vi "writeTiffFile.vi"(0 "Image Pixels (U16)":u16[][](array[numeric]), 1 "File Path":path) -> ()   [LabVIEW 2015]
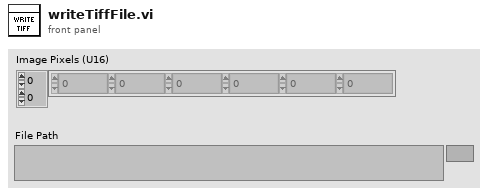
[diagram p1: front panel]
types:
  T1 = typedef "Image Type" = u32
  T2 = typedef "IMAQ Image.ctl" = refnum<image>
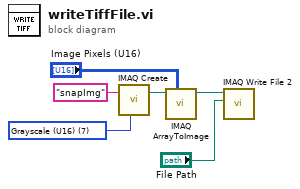
[diagram p0: block diagram]
diagram:
  w3 = T1 7 items=["Grayscale (U8)", "Grayscale (I16)", "Grayscale (SGL)", "Complex (CSG)", "RGB (U32)", "HSL (U32)", "RGB (U64)", "Grayscale (U16)"] ("Image Type")
  n1 = call "IMAQ Create"("Image Name"="snapImg", "Image Type"=w3) -> ("New Image"=w5:T2)  [unwired: 3 in, 1 out]
  n2 = call "IMAQ ArrayToImage"("Image Pixels (U16)"="Image Pixels (U16)", "Image"=w5) -> ("Image Out"=w6:T2)  [unwired: 8 in, 1 out]
  n3 = call-poly "IMAQ Write File 2"("File Path"="File Path", "Image"=w6) -> ()  [unwired: 8 in, 2 out]
